vi "radiucenterinbound.vi"(0 "Y Resolution":i32, 1 "xcenter":dbl, 2 "ycenter":dbl, 3 "Radius":dbl, 4 "X Resolution":i32) -> (5 "WithinBounds":bool)   [LabVIEW 2019]
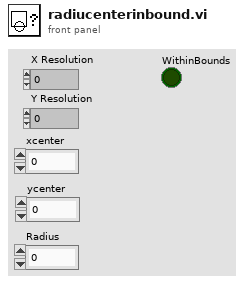
[diagram p1: front panel]
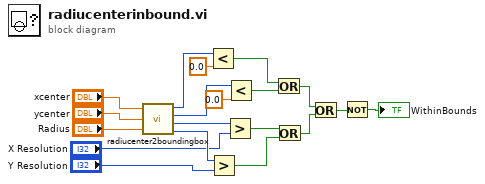
[diagram p0: block diagram]
diagram:
  n1 = call "radiucenter2boundingbox.vi"("Radius"="Radius", "ycenter"="ycenter", "xcenter"="xcenter") -> ("Bottom"=w9:i32, "Right"=w10:i32, "Top"=w13:i32, "Left"=w16:i32)  [unwired: 2 in]
  n2 = Less?(x=w16, y=0.0) -> (x < y?=w12:bool)
  n3 = Greater?(x=w9, y="Y Resolution") -> (0:w7:bool)
  n4 = Greater?(x=w10, y="X Resolution") -> (0:w8:bool)
  n5 = Less?(x=w13, y=0.0) -> (x < y?=w11:bool)
  n6 = Or(x=w12, y=w11) -> (x .or. y?=w6:bool)
  n7 = Or(x=w8, y=w7) -> (x .or. y?=w5:bool)
  n8 = Or(x=w6, y=w5) -> (x .or. y?=w4:bool)
  n9 = Not(x=w4) -> (.not. x?=→"WithinBounds":bool)
